vi "CalcExpRemainingTime.vi"(8 "error in (no error)":errorcluster, 9 "Current Dwell Time":dbl, 10 "Current Temperature":dbl, 11 "RampProgramModel in":refnum<class "RampProgramModel.lvclass">) -> (0 "error out":errorcluster, 2 "RemainExpTime(sec)":dbl, 3 "RampProgramModel out":refnum<class "RampProgramModel.lvclass">)   [LabVIEW 2015, in "RampProgramModel.lvclass"]
uses:
  RampProgramModel.lvclass
  RampProgramModel.lvclass/RampProgramModel.ctl
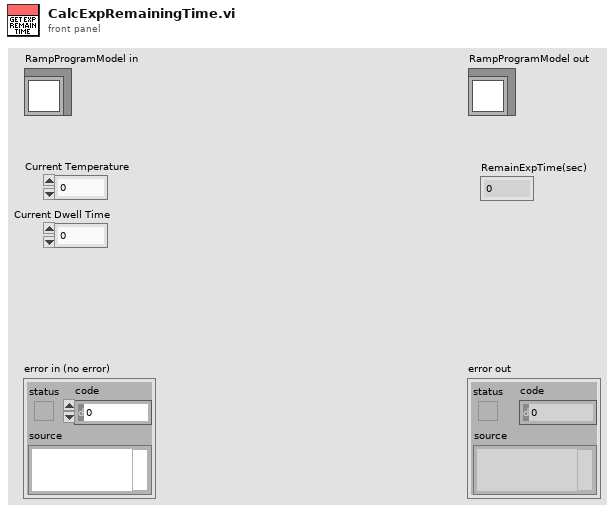
[diagram p1: front panel]
types:
  T1 = cluster{"SP (°C)":dbl, "Cooling rate (°C/min)":dbl, "Dwell Time @ SP (sec)":u32}[]
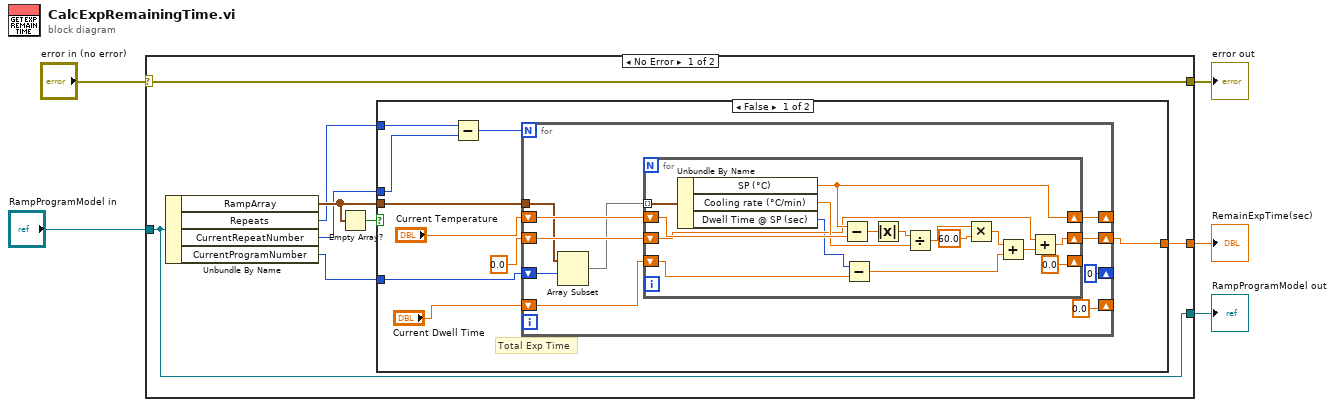
[diagram p0: block diagram]
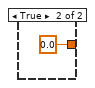
[diagram p2: hidden frame]
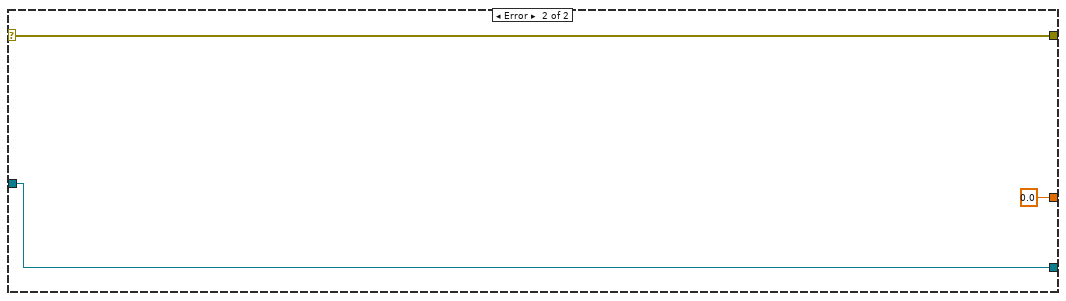
[diagram p3: hidden frame]
diagram:
  n1 = case shown="No Error" "error in (no error)" {
    selector: "error in (no error)" -> [w13 w52]
    tunnel: [w13 w52] -> w4
    tunnel: [w12 w51] -> w2
    tunnel: "RampProgramModel in" -> [w12 w51]
    tunnel: [w10 0.0 ("TotalExpTime(sec)")] -> w1
    frame No Error {
      n2 = Unbundle By Name(w12) -> ("RampArray"=w9:T1, "Repeats"=w8:u32, "CurrentRepeatNumber"=w7:u32, "CurrentProgramNumber"=w6:u32)
      n3 = Empty Array?(array=w9) -> (empty?=w11:bool)
      n4 = case shown="False" w11 {
        tunnel: [w19 0.0 ("TotalExpTime(sec)")] -> w10
        tunnel: w9 -> [w22 _]
        tunnel: w8 -> [w18 _]
        tunnel: w7 -> [w17 _]
        tunnel: w6 -> [w15 _]
        frame False {
          # "Total Exp Time"
          n5 = Subtract(x=w18, y=w17) -> (x-y=w16:u32)
          n6 = for {
            N: w16 -> [_]
            tunnel: w22 -> [w28]
            shift-right: [w30] -> w19
            shift-left: 0.0 -> [w31]
            shift-right: [w29] -> _
            shift-left: "Current Temperature" -> [w32]
            shift-right: [u32 0 ("CurrentProgramNumber")] -> _
            shift-left: w15 -> [w27]
            shift-right: [0.0 ("Current Dwell Time")] -> _
            shift-left: "Current Dwell Time" -> [w24]
            n7 = Array Subset(array=w28, index=w27) -> (w25:T1)  [unwired: 1 in]
            n8 = for {
              tunnel: w25 -> [w48] mode=indexing
              shift-right: [w40] -> w29
              shift-left: w32 -> [w47]
              shift-right: [w37] -> w30
              shift-left: w31 -> [w39]
              shift-right: [0.0 ("Current Dwell Time")] -> _
              shift-left: w24 -> [w35]
              n9 = Unbundle By Name(w48) -> ("SP (°C)"=w40:dbl, "Cooling rate (°C/min)"=w44:dbl, "Dwell Time @ SP (sec)"=w36:u32)
              n10 = Subtract(x=w40, y=w47) -> (x-y=w46:dbl)
              n11 = Subtract(x=w36, y=w35) -> (x-y=w34:dbl)
              n12 = Absolute Value(x=w46) -> (abs(x)=w45:dbl)
              n13 = Divide(x=w45, y=w44) -> (x/y=w43:dbl)
              n14 = Multiply(x=w43, y=60.0) -> (x*y=w41:dbl)
              n15 = Add(x=w41, y=w34) -> (x+y=w38:dbl)
              n16 = Add(x=w39, y=w38) -> (x+y=w37:dbl)
            }
          }
        }
        frame True {
        }
      }
    }
    frame Error {
    }
  }
  "error out" <- w4
  "RampProgramModel out" <- w2
  "RemainExpTime(sec)" <- w1
